vi "axex_read_cell.vi"(8 "error in":errorcluster, 10 "cell":T1, 11 "AX Excel instance in":T2) -> (0 "error out":errorcluster, 2 "cell string out":string, 3 "AX Excel instance out":T2)   [LabVIEW 2020, in "AX Excel.lvlib"]
doc: "Call this to read single cell. The coordinates may be given as [column,row] index or cell name such as A1, AB66, ... with priority of cell name."
uses:
  AX Excel.lvlib
  axex_instance.ctl
  axex_cell_xy.ctl
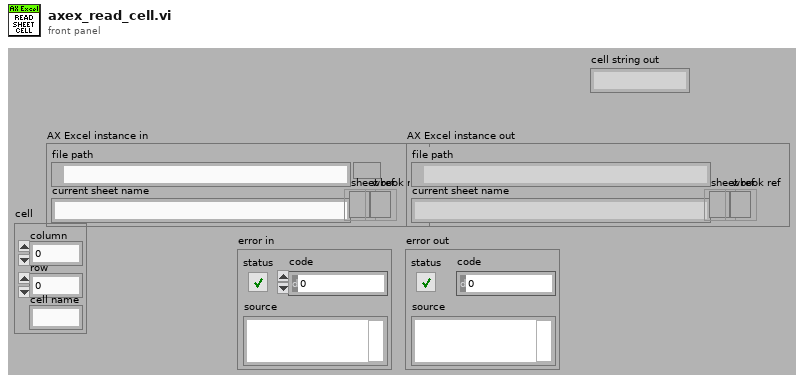
[diagram p1: front panel]
types:
  T1 = typedef "AX Excel.lvlib/axex_cell_xy.ctl" = cluster{"column":i32, "row":i32, "cell name":string}
  T2 = typedef "AX Excel.lvlib/axex_instance.ctl" = cluster{"file path":path, "current sheet name":string, "sheet ref":refnum<k7>, "wbook ref":refnum<k7>}
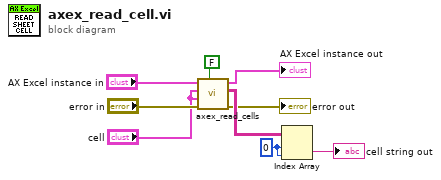
[diagram p0: block diagram]
diagram:
  w4 = 0 ("index (row)")
  n1 = call "axex_read_cells.vi"("error proof read (True)"=FALSE, "error in"="error in", "right bottom cell"="cell", "top left cell"="cell", "AX Excel instance in"="AX Excel instance in") -> ("error out"=→"error out":errorcluster, "cell array"=w5:string[][], "AX Excel instance out"=→"AX Excel instance out":T2)  [unwired: 3 in, 1 out]
  n2 = Index Array(array=w5, index (row)=w4, index (col)=w4) -> (element=→"cell string out":string)
